vi "Results to Table.vi"(6 "Result Indicators":u16[](array[numeric]), 8 "error in (no error)":errorcluster, 10 "Test Results":T1, 11 "configuration file path":path) -> (0 "error out":errorcluster, 2 "Results Table":string[][](array[string]))   [LabVIEW 2018]
panel:
  out "Pass/Fail":string[](array[string])
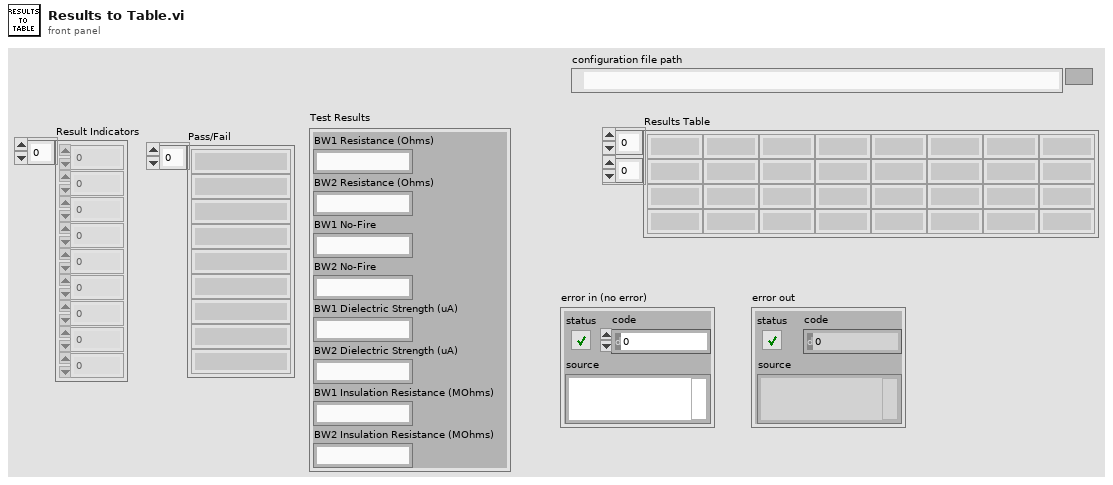
[diagram p1: front panel]
types:
  T1 = cluster{"BW1 Resistance (Ohms)":string, "BW2 Resistance (Ohms)":string, "BW1 No-Fire":string, "BW2 No-Fire":string, "BW1 Dielectric Strength (uA)":string, "BW2 Dielectric Strength (uA)":string, "BW1 Insulation Resistance (MOhms)":string, "BW2 Insulation Resistance (MOhms)":string}
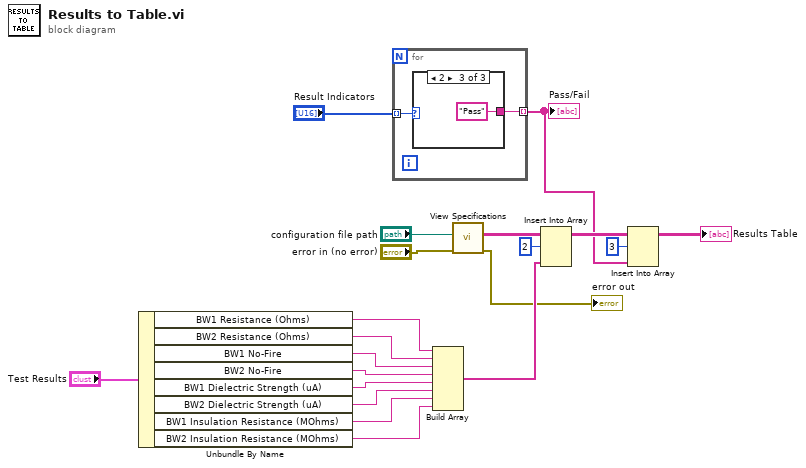
[diagram p0: block diagram]
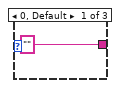
[diagram p2: hidden frame]
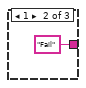
[diagram p3: hidden frame]
diagram:
  n1 = Unbundle By Name("Test Results") -> ("BW1 Resistance (Ohms)"=w18:string, "BW2 Resistance (Ohms)"=w17:string, "BW1 No-Fire"=w16:string, "BW2 No-Fire"=w15:string, "BW1 Dielectric Strength (uA)"=w14:string, "BW2 Dielectric Strength (uA)"=w13:string, "BW1 Insulation Resistance (MOhms)"=w12:string, "BW2 Insulation Resistance (MOhms)"=w11:string)
  n2 = for {
    tunnel: "Result Indicators" -> [w22] mode=indexing
    tunnel: [w21] -> w1 mode=indexing
    n3 = case shown="2" w22 {
      tunnel: ["" "Fail" "Pass"] -> w21
      frame 0, Default {
      }
      frame 1 {
      }
      frame 2 {
      }
    }
  }
  "Pass/Fail" <- w1
  n4 = Build Array(w18, w17, w16, w15, w14, w13, w12, w11) -> (w10:string[])
  n5 = call "View Specifications.vi"("error in (no error)"="error in (no error)", "configuration file path"="configuration file path") -> ("error out"=→"error out":errorcluster, "Results Table"=w8:string[][])  [unwired: 8 in]
  n6 = Insert Into Array(array=w8, index (row)=2, new element=w10) -> (w4:string[][])  [unwired: 1 in]
  n7 = Insert Into Array(array=w4, index (row)=3, new element=w1) -> (→"Results Table":string[][])  [unwired: 1 in]
